vi "sequences.vi"(0 "sequence":T4=enum."warmup", 11 "command parameter":T1={"CO2 ref"=392.0, "CO2 span"=372.0, "H2O ref"=0.0, "H2O span"=0.0, "Zi"=0.0, "Zt"=1.2, "Zm"=0.0, "S"=0.0, "Temp [C]"=50.0, "Pressure [hPa]"=135.0, "Licor-Sources"=["CO2A W", "CO2B W", "H2OA W", "H2OB W", "T C", "T V", "P kPa", "P V", "RH %", "CO2A um/m", "CO2B um/m", "H2OA mm/m", "H2OB mm/m"], "Licor-Pump"="Off", "Zeitstempel"=timestamp(0 s since 1904-01-01)} {"Pressure [hPa]" format="%.2g"; "Temp [C]" format="%.2f"; "CO2 ref" format="%.2f"; "CO2 span" format="%.2g"; "H2O ref" format="%.2g"; "H2O span" format="%.2g"}) -> (8 "sequence out":cluster{"time":i32, "command":string}[](array[cluster]))   [LabVIEW 2010]
uses:
  Licor-Sequences.ctl
  Licor-Parameter.ctl
  Licor-Steuerung/LicorLI7000/conventions/Licor-Source.ctl
  Licor-Pump.ctl
  Licor-Commands.ctl
  Licor-Steuerung/LicorLI7000/LicorLI7000.lvlib
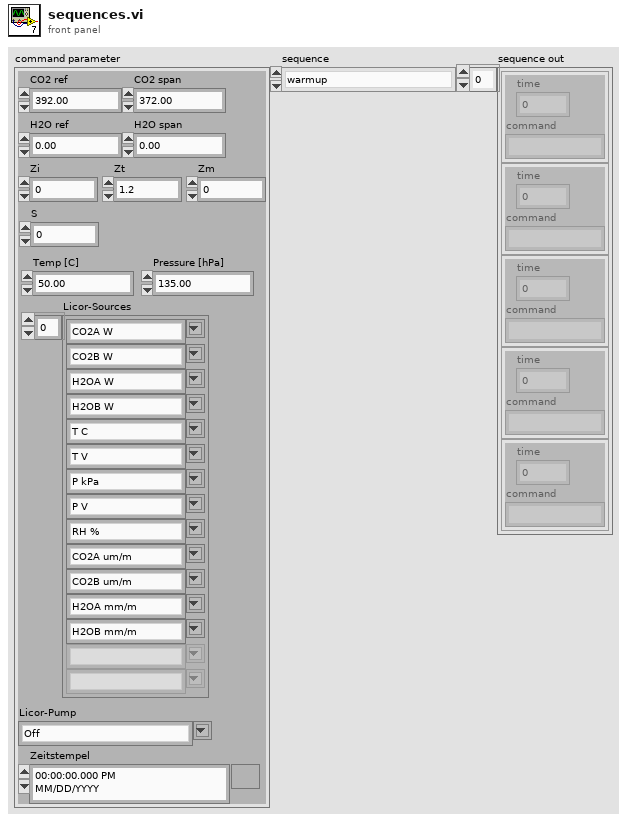
[diagram p1: front panel]
types:
  T1 = typedef "Licor-Parameter.ctl" = cluster{"CO2 ref":dbl, "CO2 span":dbl, "H2O ref":dbl, "H2O span":dbl, "Zi":dbl, "Zt":dbl, "Zm":dbl, "S":dbl, "Temp [C]":dbl, "Pressure [hPa]":dbl, "Licor-Sources":T2[], "Licor-Pump":T3, "Zeitstempel":timestamp}
  T2 = typedef "LicorLI7000.lvlib/Licor-Source.ctl" = string
  T3 = typedef "Licor-Pump.ctl" = string
  T4 = typedef "Licor-Sequences.ctl" = enum16{"test", "WAIT", "warmup", "initialize", "calibrate Z", "calibrate S"}
  T5 = typedef "Licor-Commands.ctl" = enum16{"wait", "initialize", "resetCO2", "resetH2O", "getReference", "setReference", "calibration-Z-CO2", "calibration-Z-H2O", "calibration-S-CO2", "calibration-S-H2O", "getCalibrationParameter", "setZeroParameter", "setLicorTime", "getLicorTime", "setPumpFlowrate", "setPumpSlow", "setPumpMedium", "setPumpFast", "getInfo"}
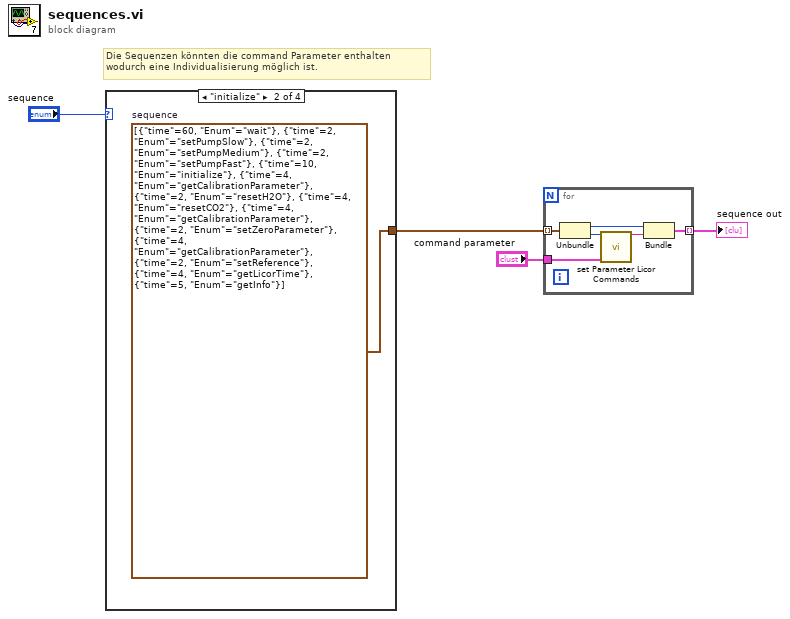
[diagram p0: block diagram]
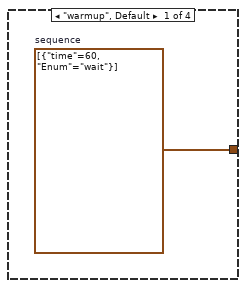
[diagram p2: hidden frame]
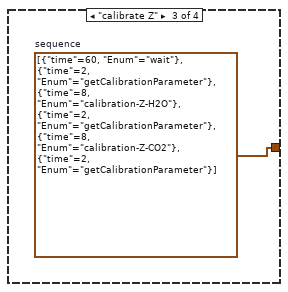
[diagram p3: hidden frame]
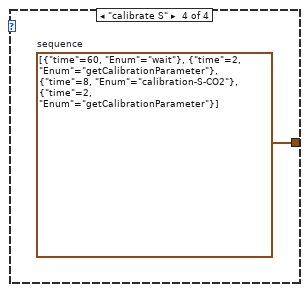
[diagram p4: hidden frame]
diagram:
  # "Die Sequenzen könnten die command Parameter enthalten \nwodurch eine Individualisierung möglich ist."
  n1 = case shown="\"initialize\"" "sequence" {
    tunnel: [w5 w6 w7 w8] -> w4
    frame "warmup", Default {
      w5 = cluster{"time":i32, "Enum":T5}[] [{"time"=60, "Enum"=enum."wait"}]  # sequence
    }
    frame "initialize" {
      w6 = cluster{"time":i32, "Enum":T5}[] [{"time"=60, "Enum"=enum."wait"}, {"time"=2, "Enum"=enum."setPumpSlow"}, {"time"=2, "Enum"=enum."setPumpMedium"}, {"time"=2, "Enum"=enum."setPumpFast"}, {"time"=10, "Enum"=enum."initialize"}, {"time"=4, "Enum"=enum."getCalibrationParameter"}, {"time"=2, "Enum"=enum."resetH2O"}, {"time"=4, "Enum"=enum."resetCO2"}, {"time"=4, "Enum"=enum."getCalibrationParameter"}, {"time"=2, "Enum"=enum."setZeroParameter"}, {"time"=4, "Enum"=enum."getCalibrationParameter"}, {"time"=2, "Enum"=enum."setReference"}, {"time"=4, "Enum"=enum."getLicorTime"}, {"time"=5, "Enum"=enum."getInfo"}]  # sequence
    }
    frame "calibrate Z" {
      w7 = cluster{"time":i32, "Enum":T5}[] [{"time"=60, "Enum"=enum."wait"}, {"time"=2, "Enum"=enum."getCalibrationParameter"}, {"time"=8, "Enum"=enum."calibration-Z-H2O"}, {"time"=2, "Enum"=enum."getCalibrationParameter"}, {"time"=8, "Enum"=enum."calibration-Z-CO2"}, {"time"=2, "Enum"=enum."getCalibrationParameter"}]  # sequence
    }
    frame "calibrate S" {
      w8 = cluster{"time":i32, "Enum":T5}[] [{"time"=60, "Enum"=enum."wait"}, {"time"=2, "Enum"=enum."getCalibrationParameter"}, {"time"=8, "Enum"=enum."calibration-S-CO2"}, {"time"=2, "Enum"=enum."getCalibrationParameter"}]  # sequence
    }
  }
  n2 = for {
    tunnel: w4 -> [w14] mode=indexing
    tunnel: "command parameter" -> [w12]
    tunnel: [w9] -> w3 mode=indexing
    n3 = Unbundle(w14) -> ("time"=w11:i32, "Enum"=w13:T5)
    n4 = call "set Parameter Licor Commands.vi"("Licor-Commands"=w13, "command parameter"=w12) -> ("command"=w10:string)  [unwired: 13 in]
    n5 = Bundle("time"=w11, "command"=w10) -> (w9:cluster{"time":i32, "command":string})  [unwired: 1 in]
  }
  "sequence out" <- w3
